vi "ER2007 Test Definition Panel.vi"() -> ()   [LabVIEW 2013]
uses:
  Controls/Global ER2007.vi
panel:
  in  "4P/2P":u16(ring) items=["2-Pole", "4-Pole"]
  in  "ZeroPore":bool
  in  "PoreXdcr":enum16{"Lo Range", "Hi Range"}(ring)
  in  "Volume Measurement":u16(ring) items=["VPA", "Manual"]
  out "NewData":bool
  in  "Stop":bool
  in  "Rw_Temp":dbl=23.0 caption="°C" min=-100.0 format="%.1f"
  in  "Rw":dbl min=0.0 format="%.3f"
  out "Cell ID":string="<none>"
  in  "DAQ Units":u16(ring) items=["Mins", "Hrs"]
  in  "File":path
  in  "Acquisition Period":dbl=60.0 min=1.0
  in  "Frequency (Hz)":dbl=1000.0 min=20.0 max=100000.0
  in  "Electrode Spacing":dbl min=0.0 format="%.3f"
  in  "Permeability":dbl format="%.1f"
  in  "Porosity":dbl format="%.1f"
  in  "Diameter":dbl min=0.0 format="%.3f"
  in  "Length":dbl min=0.0 format="%.3f"
  in  "Fluid Pair":string
  in  "Rock Type":string
  in  "Sample ID":string
  in  "Project":string
  in  "Cancel":bool
  in  "Clear":bool
  in  "Start":bool
  in  "Exit":bool
  # "Test Definition"
  # "Test Description"
  # "Sample Properties"
  # "Project"
  # "Length (cm)"
  # "Sample ID"
  # "Diameter (cm)"
  # "Rock Type"
  # "Porosity (%)"
  # "Fluid Pair"
  # "Permeability (mD)"
  # "Rw"
  # "@"
  # "Electrode Spacing (cm)"
  # "°C"
  # "Test Parameters"
  # "Frequency (Hz)"
  # "Pore Transducer"
  # "Volume Measurement"
  # "Measurement Type"
  # "File"
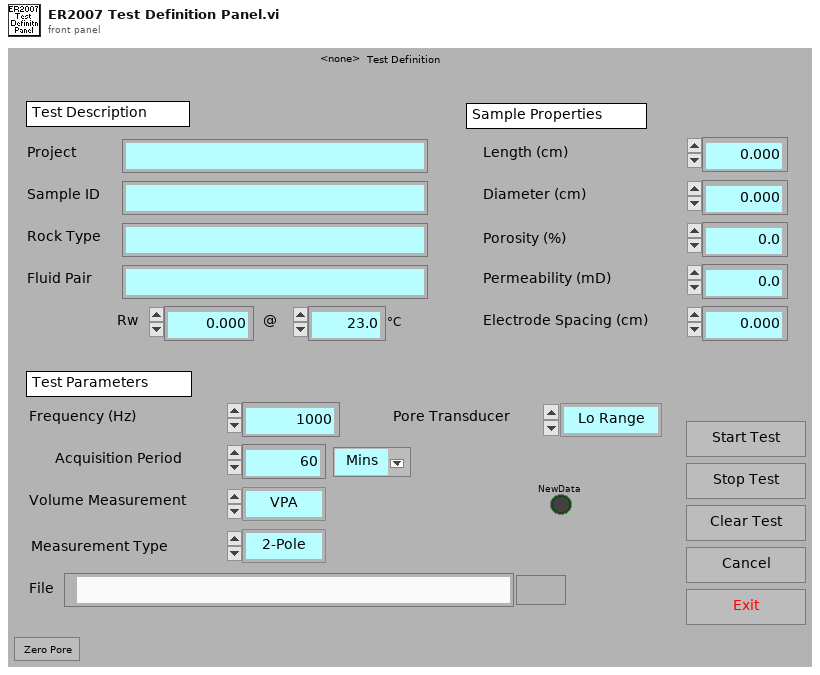
[diagram p1: front panel]
types:
  T1 = enum32{"existing file", "new file", "new or existing file", "existing dir", "new dir", "new or existing dir", "existing file (use LLBs)", "new file (use LLBs)", "new or existing file (use LLBs)", "new or existing file or directory (use LLBs)"}
  T2 = cluster{"CurCell":i32, "Cell Data":cluster{"Cell ID":i32, "Cell Status":enum16{"Inactive", "Setup", "Active", "Done"}, "Project":string, "Sample #":string, "Rock Type":string, "Fluid Pair":string, "Rw":dbl, "Rw Temp":dbl, "Length":dbl, "Diameter":dbl, "Porosity":dbl, "Permeability":dbl, "4P":bool, "ElectSpace":dbl, "Frequency":dbl, "Amplitude":dbl, "DAQ Period":u32, "DAQ Units":u16, "Start Time":dbl, "Next Time":dbl, "Datafile":path, "Last Pore Vol":dbl, "Last Pore Xdcr":enum16{"<none>", "Lo Range", "Hi Range"}, "Last Resistor":enum16{"<none>", "Resistor 1", "Resistor 2", "Resistor 3", "Resistor 4", "Resistor 5", "Resistor 6"}, "CurData":dbl[][], "Comment":string}[]}
  T3 = cluster{"Cell ID":i32, "Cell Status":enum16{"Inactive", "Setup", "Active", "Done"}, "Project":string, "Sample #":string, "Rock Type":string, "Fluid Pair":string, "Rw":dbl, "Rw Temp":dbl, "Length":dbl, "Diameter":dbl, "Porosity":dbl, "Permeability":dbl, "4P":bool, "ElectSpace":dbl, "Frequency":dbl, "Amplitude":dbl, "DAQ Period":u32, "DAQ Units":u16, "Start Time":dbl, "Next Time":dbl, "Datafile":path, "Last Pore Vol":dbl, "Last Pore Xdcr":enum16{"<none>", "Lo Range", "Hi Range"}, "Last Resistor":enum16{"<none>", "Resistor 1", "Resistor 2", "Resistor 3", "Resistor 4", "Resistor 5", "Resistor 6"}, "CurData":dbl[][], "Comment":string}[]
  T4 = cluster{"Cell ID":i32, "Cell Status":enum16{"Inactive", "Setup", "Active", "Done"}, "Project":string, "Sample #":string, "Rock Type":string, "Fluid Pair":string, "Rw":dbl, "Rw Temp":dbl, "Length":dbl, "Diameter":dbl, "Porosity":dbl, "Permeability":dbl, "4P":bool, "ElectSpace":dbl, "Frequency":dbl, "Amplitude":dbl, "DAQ Period":u32, "DAQ Units":u16, "Start Time":dbl, "Next Time":dbl, "Datafile":path, "Last Pore Vol":dbl, "Last Pore Xdcr":enum16{"<none>", "Lo Range", "Hi Range"}, "Last Resistor":enum16{"<none>", "Resistor 1", "Resistor 2", "Resistor 3", "Resistor 4", "Resistor 5", "Resistor 6"}, "CurData":dbl[][], "Comment":string}
  T5 = cluster{"PageTitle":string, "NumLines":i32, "ChlNum":string[], "ChlDesc":string[], "ChlUnits":string[], "ChlZero":sgl[], "ChlFactor":sgl[], "ChlConfig":u16[]}[]
  T6 = cluster{"PageTitle":string, "NumLines":i32, "ChlNum":string[], "ChlDesc":string[], "ChlUnits":string[], "ChlZero":sgl[], "ChlFactor":sgl[], "ChlConfig":u16[]}
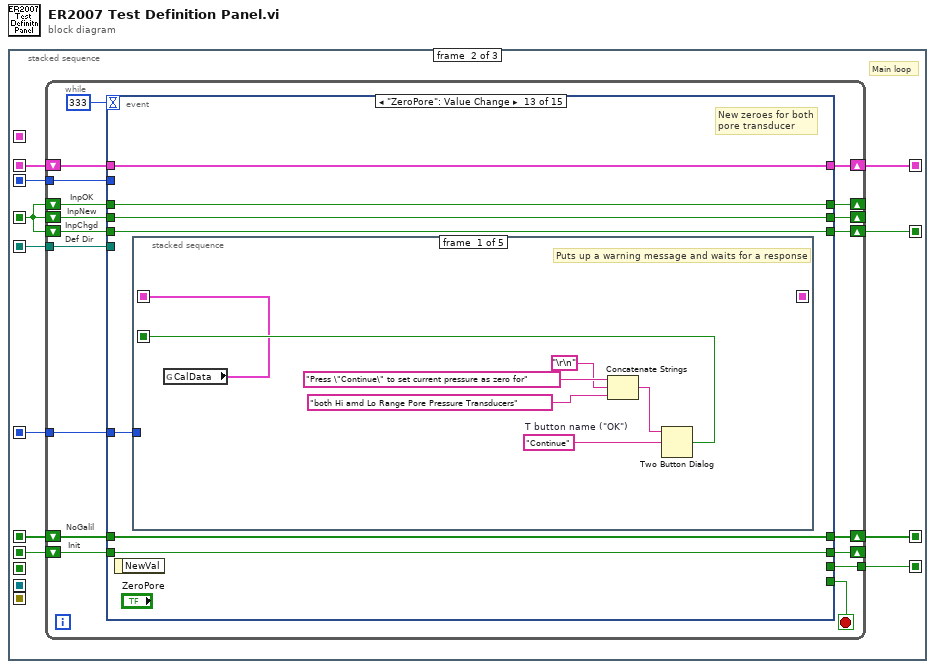
[diagram p0: block diagram]
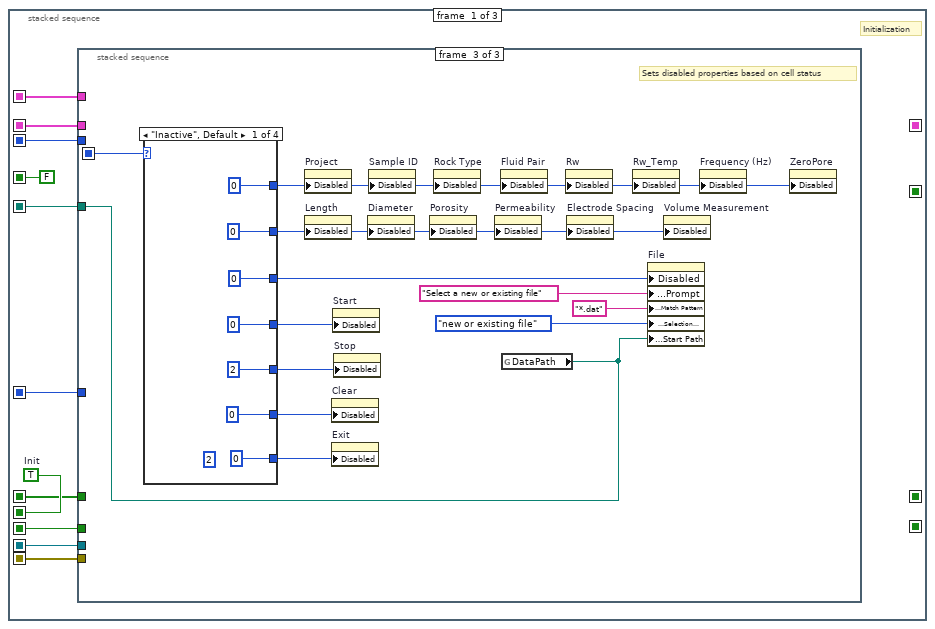
[diagram p2: hidden frame]
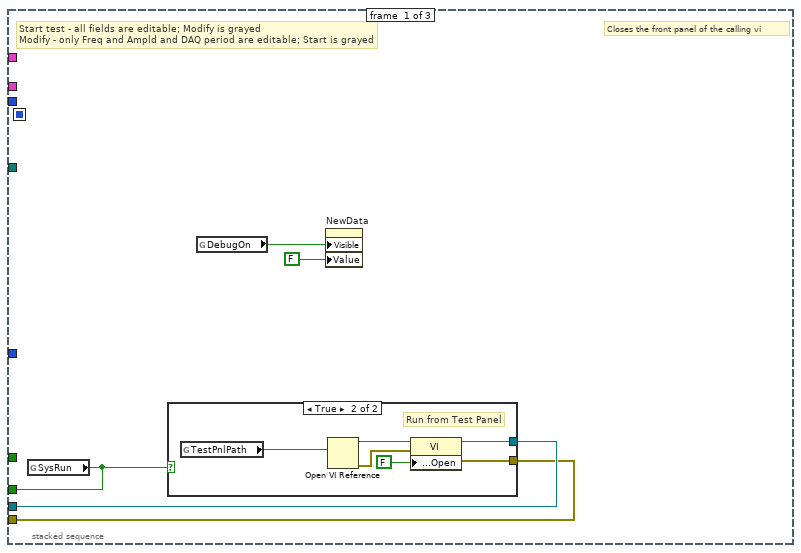
[diagram p3: hidden frame]
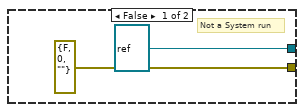
[diagram p4: hidden frame]
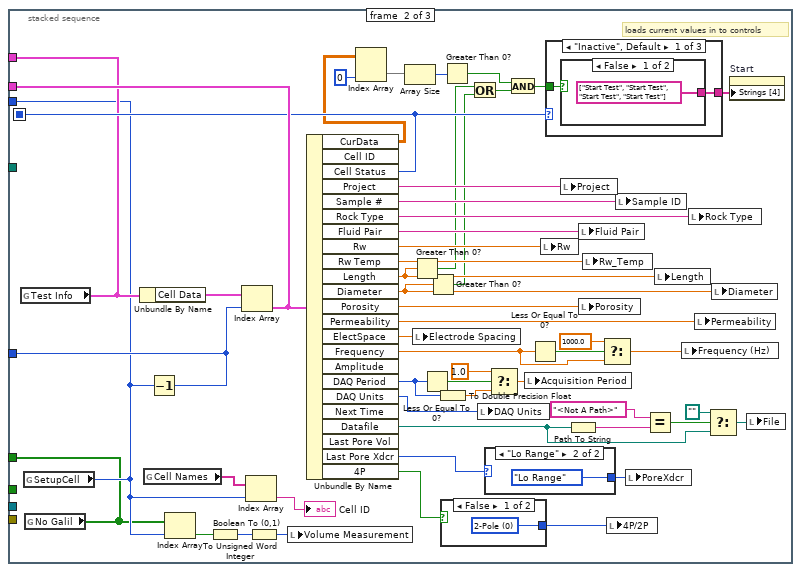
[diagram p5: hidden frame]
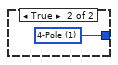
[diagram p6: hidden frame]
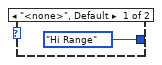
[diagram p7: hidden frame]
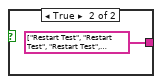
[diagram p8: hidden frame]
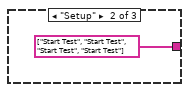
[diagram p9: hidden frame]
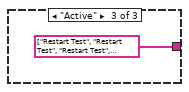
[diagram p10: hidden frame]
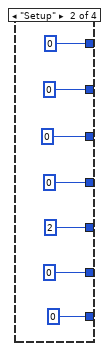
[diagram p11: hidden frame]
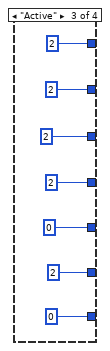
[diagram p12: hidden frame]
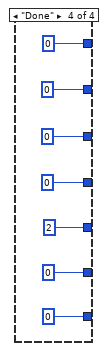
[diagram p13: hidden frame]
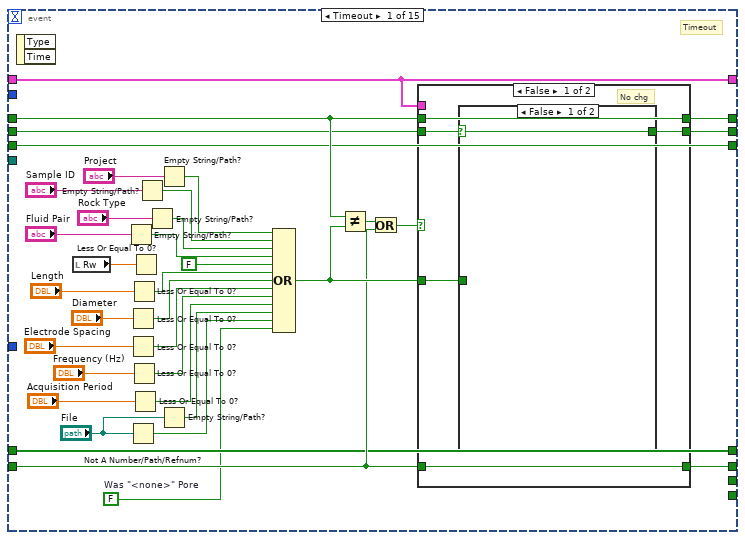
[diagram p14: hidden frame]
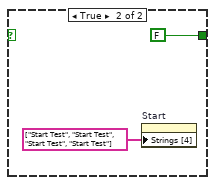
[diagram p15: hidden frame]
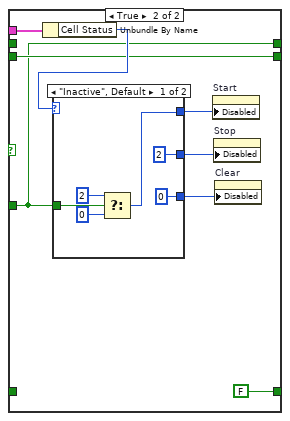
[diagram p16: hidden frame]
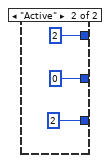
[diagram p17: hidden frame]
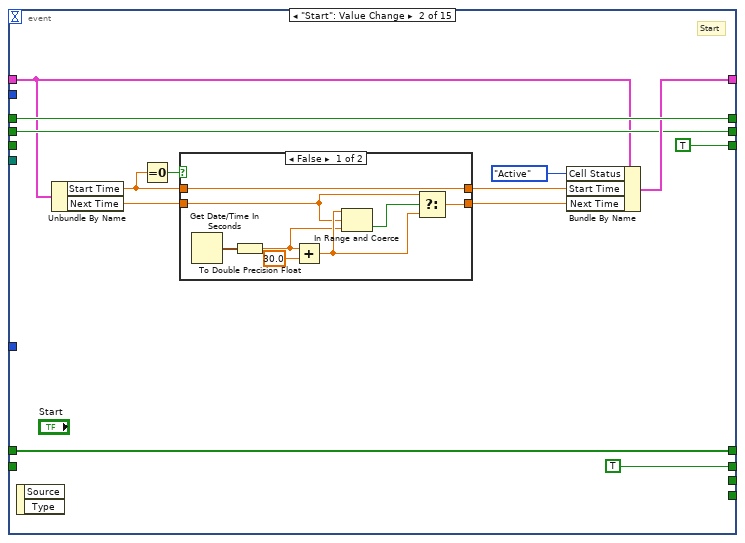
[diagram p18: hidden frame]
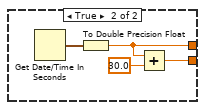
[diagram p19: hidden frame]
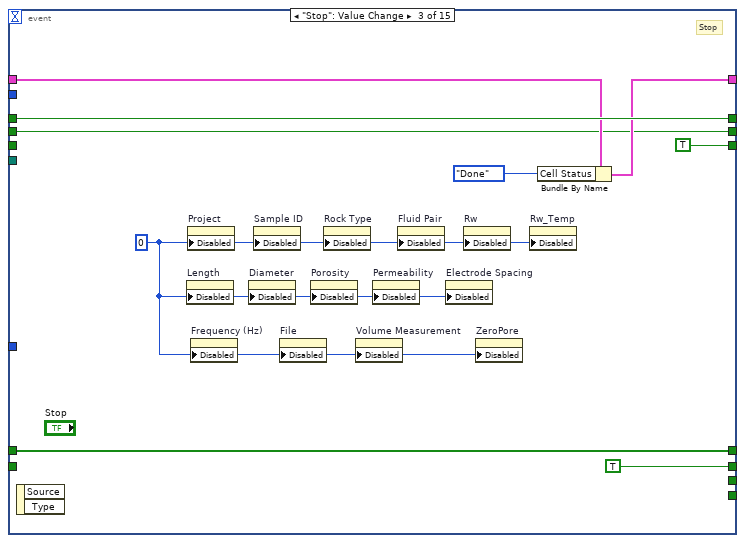
[diagram p20: hidden frame]
diagram:
  n1 = stacked-sequence {
    seq-local: [w11 _ _] -> [_ _ w495]
    seq-local: [_ w138 _] -> [_ _ w494]
    seq-local: [w10 _ _] -> [_ _ _]
    seq-local: [w9 _ _] -> [_ w136 _]
    seq-local: [w7 _ _] -> [_ w131 w493]
    seq-local: [w8 _ _] -> [_ w129 w492]
    seq-local: [w6 _ _] -> [_ _ w490]
    seq-local: [w5 _ _] -> [_ _ w491]
    seq-local: [w4 _ _] -> [_ w137 _]
    seq-local: [_ w135 _] -> [_ _ w489]
    seq-local: [_ w134 _] -> [_ _ w488]
    seq-local: [FALSE _ _] -> [_ w133 _]
    seq-local: [w2 _ _] -> [_ w132 _]
    seq-local: [w1 _ _] -> [_ w130 w487]
    seq-local: [_ w128 _] -> [_ _ w486]
    frame #0 {
      w4 = TRUE  # Init
      # "Initialization"
      n2 = stacked-sequence {
        seq-local: [_ w50 _] -> [_ _ w99]
        tunnel: [w13 _ _] -> w11
        tunnel: [_ w37 _] -> w10
        tunnel: [_ w77 _] -> w9
        tunnel: [_ w33 _] -> w8
        tunnel: [_ w34 _] -> w7
        tunnel: [w16 _ _] -> w6
        tunnel: [w15 _ _] -> w5
        tunnel: [_ _ w90] -> w2
        tunnel: [_ w29 _] -> w1
        frame #0 {
          # "Closes the front panel of the calling vi"
          # "Start test - all fields are editable; Modify is grayed\nModify - only Freq and Ampld and DAQ period are editable; Start is grayed"
          n3 = global read "Global ER2007.vi" "SysRun"() -> (w13:bool)
          n4 = case shown="True" w13 {
            tunnel: [refnum<vi> refnum w21] -> w16
            tunnel: [errorcluster {"status"=FALSE, "code"=0, "source"=""} ("error out") w20] -> w15
            frame False {
              # "Not a System run"
            }
            frame True {
              # "Run from Test Panel"
              n5 = global read "Global ER2007.vi" "TestPnlPath"() -> (w19:path)
              n6 = Open VI Reference(vi path=w19) -> (vi reference=w24:refnum<vi>, error out=w23:errorcluster)  [unwired: 5 in]
              n7 = property class="VI"(reference=w24, error in=w23, "Front Panel Window:Open"=FALSE) -> (reference out=w21:refnum<vi>, error out=w20:errorcluster)
            }
          }
          n8 = global read "Global ER2007.vi" "DebugOn"() -> (w12:bool)
          n9 = property on="NewData" class="Bool (strict)"("Visible"=w12, "Value"=FALSE ("NewData")) -> ()  [unwired: 2 in, 2 out]
        }
        frame #1 {
          # "loads current values in to controls"
          n10 = global read "Global ER2007.vi" "Test Info"() -> (w37:T2)
          n11 = global read "Global ER2007.vi" "SetupCell"() -> (w33:i32)
          n12 = global read "Global ER2007.vi" "No Galil"() -> (w29:bool[])
          n13 = Unbundle By Name(w37) -> ("Cell Data"=w68:T3)
          n14 = global read "Global ER2007.vi" "Cell Names"() -> (w36:string[])
          n15 = Decrement(x=w33) -> (x-1=w34:i32)
          n16 = Index Array(array=w29, index=w33) -> (element=w32:bool)
          n17 = Boolean To (0,1)(Boolean=w32) -> (0, 1=w31:i16)
          n18 = Index Array(array=w68, index=w34) -> (element=w77:T4)
          n19 = Index Array(array=w36, index=w33) -> (element=→"Cell ID":string)
          n20 = To Unsigned Word Integer(number=w31) -> (unsigned 16bit integer=w30:u16)
          n21 = local write "Volume Measurement"(w30) -> ()
          n22 = Unbundle By Name(w77) -> ("CurData"=w44:dbl[][], "Cell Status"=w50:enum16{"Inactive", "Setup", "Active", "Done"}, "Project"=w76:string, "Sample #"=w75:string, "Rock Type"=w74:string, "Fluid Pair"=w73:string, "Rw"=w67:dbl, "Rw Temp"=w66:dbl, "Length"=w48:dbl, "Diameter"=w47:dbl, "Porosity"=w72:dbl, "Permeability"=w71:dbl, "ElectSpace"=w70:dbl, "Frequency"=w59:dbl, "DAQ Period"=w65:u32, "DAQ Units"=w69:u16, "Datafile"=w53:path, "Last Pore Xdcr"=w27:enum16{"<none>", "Lo Range", "Hi Range"}, "4P"=w26:bool)  [unwired: 4 out]
          n23 = Index Array(array=w44, index (col)=0 ("disabled index (col)")) -> (element=w42:dbl[])  [unwired: 1 in]
          n24 = Array Size(array=w42) -> (size(s)=w39:i32)
          n25 = Greater Than 0?(x=w48) -> (x > 0?=w46:bool)
          n26 = local write "Electrode Spacing"(w70) -> ()
          n27 = Less Or Equal To 0?(x=w65) -> (x <= 0?=w64:bool)
          n28 = Greater Than 0?(x=w47) -> (x > 0?=w45:bool)
          n29 = To Double Precision Float(number=w65) -> (double precision float=w63:dbl)
          n30 = case shown="False" w26 {
            tunnel: [w78 w79] -> w25
            frame False {
              w78 = u16 0 items=["2-Pole", "4-Pole"] ("4P/2P")
            }
            frame True {
              w79 = u16 1 items=["2-Pole", "4-Pole"] ("4P/2P")
            }
          }
          n31 = Greater Than 0?(x=w39) -> (x > 0?=w38:bool)
          n32 = Or(x=w46, y=w45) -> (x .or. y?=w40:bool)
          n33 = local write "DAQ Units"(w69) -> ()
          n34 = case shown="\"Lo Range\"" w27 {
            tunnel: [enum16{"Lo Range", "Hi Range"}."Hi Range" ("PoreXdcr") enum16{"Lo Range", "Hi Range"}."Lo Range" ("PoreXdcr")] -> w28
            frame "<none>", Default {
            }
            frame "Lo Range" {
            }
          }
          n35 = Select(t=1.0, s=w64, f=w63) -> (s? t:f=w62:dbl)
          n36 = And(x=w38, y=w40) -> (x .and. y?=w41:bool)
          n37 = local write "Acquisition Period"(w62) -> ()
          n38 = Less Or Equal To 0?(x=w59) -> (x <= 0?=w60:bool)
          n39 = local write "Rw"(w67) -> ()
          n40 = case shown="\"Inactive\", Default" w50 {
            tunnel: [w83 string[] ["Start Test", "Start Test", "Start Test", "Start Test"] ("Strings [4]") string[] ["Restart Test", "Restart Test", "Restart Test", "Restart Test"] ("Strings [4]")] -> w49
            tunnel: w41 -> [w82 _ _]
            frame "Inactive", Default {
              n41 = case shown="False" w82 {
                tunnel: [string[] ["Start Test", "Start Test", "Start Test", "Start Test"] ("Strings [4]") string[] ["Restart Test", "Restart Test", "Restart Test", "Restart Test"] ("Strings [4]")] -> w83
                frame False {
                }
                frame True {
                }
              }
            }
            frame "Setup" {
            }
            frame "Active" {
            }
          }
          n42 = local write "Project"(w76) -> ()
          n43 = Path To String(path=w53) -> (string=w55:string)
          n44 = local write "Fluid Pair"(w73) -> ()
          n45 = local write "Porosity"(w72) -> ()
          n46 = local write "Rw_Temp"(w66) -> ()
          n47 = Select(t=1000.0, s=w60, f=w59) -> (s? t:f=w58:dbl)
          n48 = local write "4P/2P"(w25) -> ()
          n49 = local write "Sample ID"(w75) -> ()
          n50 = local write "PoreXdcr"(w28) -> ()
          n51 = Equal?(x="<Not A Path>" ("y"), y=w55) -> (x = y?=w56:bool)
          n52 = local write "Length"(w48) -> ()
          n53 = local write "Frequency (Hz)"(w58) -> ()
          n54 = local write "Rock Type"(w74) -> ()
          n55 = local write "Permeability"(w71) -> ()
          n56 = Select(t=path "", s=w56, f=w53) -> (s? t:f=w52:path)
          n57 = local write "Diameter"(w47) -> ()
          n58 = property on="Start" class="Bool"("Strings [4]"=w49) -> ()  [unwired: 2 in, 2 out]
          n59 = local write "File"(w52) -> ()
        }
        frame #2 {
          # "Sets disabled properties based on cell status"
          n60 = case shown="\"Inactive\", Default" w99 {
            tunnel: [u8 0 ("Disabled") u8 0 ("Disabled") u8 2 ("Disabled") u8 0 ("Disabled")] -> w89
            tunnel: [u8 0 ("Disabled") u8 0 ("Disabled") u8 2 ("Disabled") u8 0 ("Disabled")] -> w88
            tunnel: [u8 0 ("Disabled") u8 0 ("Disabled") u8 2 ("Disabled") u8 0 ("Disabled")] -> w98
            tunnel: [u8 0 ("Disabled") u8 0 ("Disabled") u8 2 ("Disabled") u8 0 ("Disabled")] -> w97
            tunnel: [u8 0 ("Disabled") u8 0 ("Disabled") u8 2 ("Disabled") u8 0 ("Disabled")] -> w96
            tunnel: [u8 2 ("Disabled") u8 2 ("Disabled") u8 0 ("Disabled") u8 2 ("Disabled")] -> w95
            tunnel: [u8 0 ("Disabled") u8 0 ("Disabled") u8 0 ("Disabled") u8 0 ("Disabled")] -> w94
            frame "Inactive", Default {
              (unwired) u8 2 ("Disabled")
            }
            frame "Setup" {
            }
            frame "Active" {
            }
            frame "Done" {
            }
          }
          n61 = property on="Project" class="Str"("Disabled"=w89) -> ()  [unwired: 2 in, 2 out]
          n62 = property on="Length" class="DigNum (strict)"("Disabled"=w88) -> ()  [unwired: 2 in, 2 out]
          n63 = property on="Clear" class="Bool"("Disabled"=w97) -> ()  [unwired: 2 in, 2 out]
          n64 = property on="Exit" class="Bool"("Disabled"=w94) -> ()  [unwired: 2 in, 2 out]
          n65 = property on="Start" class="Bool"("Disabled"=w98) -> ()  [unwired: 2 in, 2 out]
          n66 = property on="Stop" class="Bool"("Disabled"=w95) -> ()  [unwired: 2 in, 2 out]
          n67 = property on="Diameter" class="DigNum (strict)"("Disabled"=w88) -> ()  [unwired: 2 in, 2 out]
          n68 = property on="Sample ID" class="Str"("Disabled"=w89) -> ()  [unwired: 2 in, 2 out]
          n69 = property on="Porosity" class="DigNum (strict)"("Disabled"=w88) -> ()  [unwired: 2 in, 2 out]
          n70 = property on="Rock Type" class="Str"("Disabled"=w89) -> ()  [unwired: 2 in, 2 out]
          n71 = property on="Permeability" class="DigNum (strict)"("Disabled"=w88) -> ()  [unwired: 2 in, 2 out]
          n72 = property on="Fluid Pair" class="Str"("Disabled"=w89) -> ()  [unwired: 2 in, 2 out]
          n73 = global read "Global ER2007.vi" "DataPath"() -> (w90:path)
          n74 = property on="Rw" class="DigNum (strict)"("Disabled"=w89) -> ()  [unwired: 2 in, 2 out]
          n75 = property on="Electrode Spacing" class="DigNum (strict)"("Disabled"=w88) -> ()  [unwired: 2 in, 2 out]
          n76 = property on="Rw_Temp" class="DigNum (strict)"("Disabled"=w89) -> ()  [unwired: 2 in, 2 out]
          n77 = property on="File" class="Path"("Disabled"=w96, "Browse Options:Prompt"="Select a new or existing file" ("Browse Dialog Options:Prompt"), "Browse Options:Match Pattern"="*.dat" ("Browse Dialog Options:Match Pattern"), "Browse Options:Selection Mode"=T1."new or existing file" ("Browse Dialog Options:Selection Mode"), "Browse Options:Start Path"=w90) -> ()  [unwired: 2 in, 2 out]
          n78 = property on="Volume Measurement" class="Ring (strict)"("Disabled"=w88) -> ()  [unwired: 2 in, 2 out]
          n79 = property on="Frequency (Hz)" class="DigNum (strict)"("Disabled"=w89) -> ()  [unwired: 2 in, 2 out]
          n80 = property on="ZeroPore" class="Bool"("Disabled"=w89) -> ()  [unwired: 2 in, 2 out]
        }
      }
    }
    frame #1 {
      # "Main loop"
      n81 = while {
        tunnel: [w154] -> w138
        shift-right: [w152] -> _
        shift-left: w133 -> [w153]
        shift-right: [w150] -> _
        shift-left: w137 -> [w151]
        shift-right: [w148] -> w135
        shift-left: w136 -> [w149]
        shift-right: [w146] -> _
        shift-left: w133 -> [w147]
        shift-right: [w144] -> w134
        shift-left: w133 -> [w145]
        tunnel: w132 -> [w143]
        tunnel: w131 -> [w142]
        shift-right: [w140] -> w128
        shift-left: w130 -> [w141]
        tunnel: w129 -> [w139]
        stop <- w155 stop-if-true
        # "Init"
        # "NoGalil"
        # "Def Dir"
        # "InpNew"
        # "InpOK"
        # "InpChgd"
        n82 = event shown="[12] \"ZeroPore\": Value Change" {
          selector: _ -> [_ _ _ _ _ _ _ _ _ _ _ _ _ _ _]
          dyn-events: _ -> [_ _ _ _ _ _ _ _ _ _ _ _ _ _ _]
          timeout: 333 -> [_ _ _ _ _ _ _ _ _ _ _ _ _ _ _]
          tunnel: [_ _ _ _ _ _ _ _ _ _ _ _ _ w460 w464] -> w155
          tunnel: [_ _ _ _ _ _ _ _ _ _ _ _ _ FALSE w464] -> w154
          tunnel: w153 -> [w185 w230 w251 w274 w281 w287 w294 w299 w309 w315 w337 w381 w389 w458 w465]
          tunnel: [w183 w230 w251 w274 w281 w287 w294 w299 w309 w315 w337 w381 w389 w458 w465] -> w152
          tunnel: w151 -> [w162 _ _ _ w279 w285 w291 w296 w307 w311 w339 w377 w385 w457 w468]
          tunnel: [w163 TRUE ("Init") TRUE ("Init") TRUE ("Init") w279 w285 w291 w296 w307 w311 w339 w377 w385 w457 w468] -> w150
          tunnel: w149 -> [w181 w223 w249 _ w282 w288 w293 w300 w310 w316 w338 w382 w384 w456 w467]
          tunnel: [w181 w228 w248 w256 w282 w288 w293 w300 w310 w316 w338 w382 w384 w456 w467] -> w148
          tunnel: w147 -> [w161 w224 w246 _ _ _ _ w298 _ _ _ w380 w388 w455 w466]
          tunnel: [w160 w224 w246 TRUE TRUE TRUE TRUE w298 TRUE FALSE TRUE w380 w388 w455 w466] -> w146
          tunnel: w145 -> [w159 _ _ _ _ _ _ _ _ _ _ _ w387 _ w463]
          tunnel: [w159 TRUE TRUE TRUE TRUE TRUE TRUE TRUE TRUE TRUE TRUE TRUE w387 FALSE w463] -> w144
          tunnel: w143 -> [_ _ _ _ _ _ _ _ _ _ w322 _ _ _ _]
          tunnel: w142 -> [_ _ _ _ _ _ _ _ _ _ w318 _ w383 _ _]
          tunnel: w141 -> [w158 w218 w244 w253 w277 w283 w289 w295 w306 w312 w317 w378 w386 w453 w461]
          tunnel: [w158 w218 w244 w253 w277 w283 w289 w295 w305 w312 w317 w378 w386 w453 w461] -> w140
          tunnel: w139 -> [_ _ _ _ _ _ _ _ w304 _ _ _ _ _ _]
          event Timeout {
            w157 = FALSE  # Was "<none>" Pore
            # "Timeout"
            n83 = event-data() -> ()  [unwired: 1 in, 2 out]
            n84 = local read "Rw"() -> (w164:dbl)
            n85 = Empty String/Path?(string/path="Fluid Pair") -> (empty?=w189:bool)
            n86 = Less Or Equal To 0?(x="Diameter") -> (x <= 0?=w187:bool)
            n87 = Less Or Equal To 0?(x="Electrode Spacing") -> (x <= 0?=w186:bool)
            n88 = Not A Number/Path/Refnum?(number/path/refnum="File") -> (NaN/Path/Refnum?=w179:bool)
            n89 = Less Or Equal To 0?(x="Length") -> (x <= 0?=w188:bool)
            n90 = Less Or Equal To 0?(x="Frequency (Hz)") -> (x <= 0?=w177:bool)
            n91 = Less Or Equal To 0?(x="Acquisition Period") -> (x <= 0?=w168:bool)
            n92 = Less Or Equal To 0?(x=w164) -> ()  [unwired: 1 out]
            n93 = Empty String/Path?(string/path="Sample ID") -> (empty?=w191:bool)
            n94 = Empty String/Path?(string/path="Rock Type") -> (empty?=w190:bool)
            n95 = Empty String/Path?(string/path="Project") -> (empty?=w192:bool)
            n96 = Empty String/Path?(string/path="File") -> (empty?=w178:bool)
            n97 = Compound Arithmetic op=OR(w192, w191, w190, w189, FALSE ("value"), w188, w187, w186, w177, w168, w178, w179, w157) -> (w180:bool)
            n98 = Not Equal?(x=w185, y=w180) -> (x != y?=w184:bool)
            n99 = Or(x=w184, y=w162) -> (x .or. y?=w182:bool)
            n100 = case shown="False" w182 {
              tunnel: w185 -> [w197 _]
              tunnel: [w197 w201] -> w183
              tunnel: w180 -> [w193 w201]
              tunnel: w181 -> [_ w208]
              tunnel: [w196 FALSE ("Init")] -> w163
              tunnel: w162 -> [w196 _]
              tunnel: w161 -> [w195 w202]
              tunnel: [w194 w202] -> w160
              frame False {
                # "No chg"
                n101 = case shown="False" w195 {
                  selector: w195 -> [w198 _]
                  tunnel: [w198 FALSE] -> w194
                  tunnel: w193 -> [_ _]
                  frame False {
                  }
                  frame True {
                    n102 = property on="Start" class="Bool"("Strings [4]"=string[] ["Start Test", "Start Test", "Start Test", "Start Test"]) -> ()  [unwired: 2 in, 2 out]
                  }
                }
              }
              frame True {
                n103 = Unbundle By Name(w208) -> ("Cell Status"=w207:enum16{"Inactive", "Setup", "Active", "Done"})
                n104 = case shown="\"Inactive\", Default" w207 {
                  tunnel: [u8 2 ("Disabled") u8 0 ("Disabled")] -> w206
                  tunnel: [w209 u8 2 ("Disabled")] -> w205
                  tunnel: [u8 0 ("Disabled") u8 2 ("Disabled")] -> w204
                  tunnel: w201 -> [w210 _]
                  frame "Inactive", Default {
                    n105 = Select(t=u8 2 ("Disabled"), s=w210, f=u8 0 ("Disabled")) -> (s? t:f=w209:u8)
                  }
                  frame "Active" {
                  }
                }
                n106 = property on="Start" class="Bool"("Disabled"=w205) -> ()  [unwired: 2 in, 2 out]
                n107 = property on="Stop" class="Bool"("Disabled"=w206) -> ()  [unwired: 2 in, 2 out]
                n108 = property on="Clear" class="Bool"("Disabled"=w204) -> ()  [unwired: 2 in, 2 out]
              }
            }
          }
          event "Start": Value Change {
            # "Start"
            n109 = event-data() -> ()  [unwired: 1 in, 2 out]
            n110 = Unbundle By Name(w223) -> ("Start Time"=w221:dbl, "Next Time"=w222:dbl)
            n111 = Equal To 0?(x=w221) -> (x = 0?=w219:bool)
            n112 = case shown="False" w219 {
              tunnel: [w236 w240] -> w226
              tunnel: [w238 w239] -> w225
              tunnel: w222 -> [w232 _]
              tunnel: w221 -> [w238 _]
              frame False {
                n113 = Get Date/Time In Seconds() -> (seconds since 1Jan1904=w237:timestamp)
                n114 = To Double Precision Float(number=w237) -> (double precision float=w233:dbl)
                n115 = Add(x=w233, y=30.0) -> (x+y=w234:dbl)
                n116 = In Range and Coerce(upper limit=w234, x=w232, lower limit=w233) -> (In Range?=w231:bool)  [unwired: 1 out]
                n117 = Select(t=w232, s=w231, f=w234) -> (s? t:f=w236:dbl)
              }
              frame True {
                n118 = Get Date/Time In Seconds() -> (seconds since 1Jan1904=w242:timestamp)
                n119 = To Double Precision Float(number=w242) -> (double precision float=w239:dbl)
                n120 = Add(x=w239, y=30.0) -> (x+y=w240:dbl)
              }
            }
            n121 = Bundle By Name(cluster=w223, "Cell Status"=enum16{"Inactive", "Setup", "Active", "Done"}."Active", "Start Time"=w225, "Next Time"=w226) -> (w228:T4)
          }
          event "Stop": Value Change {
            w243 = u8 0 ("Disabled")
            # "Stop"
            n122 = event-data() -> ()  [unwired: 1 in, 2 out]
            n123 = property on="Length" class="DigNum (strict)"("Disabled"=w243) -> ()  [unwired: 2 in, 2 out]
            n124 = property on="Project" class="Str"("Disabled"=w243) -> ()  [unwired: 2 in, 2 out]
            n125 = property on="Frequency (Hz)" class="DigNum (strict)"("Disabled"=w243) -> ()  [unwired: 2 in, 2 out]
            n126 = property on="Diameter" class="DigNum (strict)"("Disabled"=w243) -> ()  [unwired: 2 in, 2 out]
            n127 = property on="Sample ID" class="Str"("Disabled"=w243) -> ()  [unwired: 2 in, 2 out]
            n128 = property on="File" class="Path"("Disabled"=w243) -> ()  [unwired: 2 in, 2 out]
            n129 = property on="Porosity" class="DigNum (strict)"("Disabled"=w243) -> ()  [unwired: 2 in, 2 out]
            n130 = property on="Rock Type" class="Str"("Disabled"=w243) -> ()  [unwired: 2 in, 2 out]
            n131 = property on="Volume Measurement" class="Ring (strict)"("Disabled"=w243) -> ()  [unwired: 2 in, 2 out]
            n132 = property on="Permeability" class="DigNum (strict)"("Disabled"=w243) -> ()  [unwired: 2 in, 2 out]
            n133 = property on="Fluid Pair" class="Str"("Disabled"=w243) -> ()  [unwired: 2 in, 2 out]
            n134 = property on="Electrode Spacing" class="DigNum (strict)"("Disabled"=w243) -> ()  [unwired: 2 in, 2 out]
            n135 = property on="Rw" class="DigNum (strict)"("Disabled"=w243) -> ()  [unwired: 2 in, 2 out]
            n136 = property on="ZeroPore" class="Bool"("Disabled"=w243) -> ()  [unwired: 2 in, 2 out]
            n137 = property on="Rw_Temp" class="DigNum (strict)"("Disabled"=w243) -> ()  [unwired: 2 in, 2 out]
            n138 = Bundle By Name(cluster=w249, "Cell Status"=enum16{"Inactive", "Setup", "Active", "Done"}."Done") -> (w248:T4)
          }
          event "Clear": Value Change {
            w256 = T4 {"Cell ID"=0, "Cell Status"=enum."Inactive", "Project"="", "Sample #"="", "Rock Type"="", "Fluid Pair"="", "Rw"=0.0, "Rw Temp"=0.0, "Length"=0.0, "Diameter"=0.0, "Porosity"=0.0, "Permeability"=0.0, "4P"=TRUE, "ElectSpace"=0.0, "Frequency"=0.0, "Amplitude"=0.0, "DAQ Period"=0, "DAQ Units"=0, "Start Time"=0.0, "Next Time"=0.0, "Datafile"=path "", "Last Pore Vol"=0.0, "Last Pore Xdcr"=enum."<none>", "Last Resistor"=enum."<none>", "CurData"=[], "Comment"=""} ("Cell x Data")
            w255 = u8 0 ("Disabled")
            # "Clear"
            n139 = event-data() -> ()  [unwired: 1 in, 2 out]
            n140 = Unbundle By Name(w256) -> ("Project"=w272:string, "Sample #"=w271:string, "Rock Type"=w270:string, "Fluid Pair"=w269:string, "Rw"=w268:dbl, "Rw Temp"=w267:dbl, "Length"=w266:dbl, "Diameter"=w265:dbl, "Porosity"=w264:dbl, "Permeability"=w263:dbl, "ElectSpace"=w262:dbl, "Datafile"=w259:path, "4P"=w254:bool)
            n141 = case shown="False" w254 {
              tunnel: [w275 w276] -> w252
              frame False {
                w275 = u16 0 items=["2-Pole", "4-Pole"] ("4P/2P")
              }
              frame True {
                w276 = u16 1 items=["2-Pole", "4-Pole"] ("4P/2P")
              }
            }
            n142 = global write "Global ER2007.vi" "SUP Cleared"(TRUE ("SUP Cleared")) -> ()
            n143 = local write "4P/2P"(w252) -> ()
            n144 = property on="Project" class="Str"("Disabled"=w255, "Value"=w272) -> ()  [unwired: 2 in, 2 out]
            n145 = property on="Rw" class="DigNum (strict)"("Disabled"=w255, "Value"=w268) -> ()  [unwired: 2 in, 2 out]
            n146 = property on="Porosity" class="DigNum (strict)"("Disabled"=w255, "Value"=w264) -> ()  [unwired: 2 in, 2 out]
            n147 = property on="Permeability" class="DigNum (strict)"("Disabled"=w255, "Value"=w263) -> ()  [unwired: 2 in, 2 out]
            n148 = property on="Rw_Temp" class="DigNum (strict)"("Disabled"=w255, "Value"=w267) -> ()  [unwired: 2 in, 2 out]
            n149 = property on="File" class="Path"("Disabled"=w255, "Value"=w259) -> ()  [unwired: 2 in, 2 out]
            n150 = property on="Sample ID" class="Str"("Disabled"=w255, "Value"=w271) -> ()  [unwired: 2 in, 2 out]
            n151 = property on="Volume Measurement" class="Ring (strict)"("Disabled"=w255) -> ()  [unwired: 2 in, 2 out]
            n152 = property on="Length" class="DigNum (strict)"("Disabled"=w255, "Value"=w266) -> ()  [unwired: 2 in, 2 out]
            n153 = property on="Electrode Spacing" class="DigNum (strict)"("Disabled"=w255, "Value"=w262) -> ()  [unwired: 2 in, 2 out]
            n154 = property on="Rock Type" class="Str"("Disabled"=w255, "Value"=w270) -> ()  [unwired: 2 in, 2 out]
            n155 = property on="ZeroPore" class="Bool"("Disabled"=w255) -> ()  [unwired: 2 in, 2 out]
            n156 = property on="Frequency (Hz)" class="DigNum (strict)"("Disabled"=w255, "Value"=1000.0 ("Frequency (Hz)")) -> ()  [unwired: 2 in, 2 out]
            n157 = property on="Fluid Pair" class="Str"("Disabled"=w255, "Value"=w269) -> ()  [unwired: 2 in, 2 out]
            n158 = property on="Diameter" class="DigNum (strict)"("Disabled"=w255, "Value"=w265) -> ()  [unwired: 2 in, 2 out]
          }
          event "Project", "Sample ID", "Rock Type", "Fluid Pair", "Rw", "Rw_Temp": Value Change {
            # "Project, etc"
            n159 = event-data() -> ()  [unwired: 1 in, 2 out]
          }
          event "Length", "Diameter", "Porosity", "Permeability", "Electrode Spacing": Value Change {
            # "Length, etc"
            n160 = event-data() -> ()  [unwired: 1 in, 2 out]
          }
          event "Frequency (Hz)": Value Change {
            # "Frequency chgd"
            n161 = event-data() -> ()  [unwired: 1 in, 2 out]
          }
          event "Acquisition Period": Value Change {
            # "Acquisition period chgd"
            n162 = event-data() -> ()  [unwired: 1 in, 2 out]
          }
          event "Volume Measurement": Value Change {
            # "Vol Measurement chgd"
            n163 = event-data() -> ()  [unwired: 1 in, 2 out]
            n164 = Not Equal To 0?(x="Volume Measurement") -> (x != 0?=w302:bool)
            n165 = Replace Array Subset(array=w306, new element=w302, index=w304) -> (w305:bool[])
          }
          event "4P/2P": Value Change {
            # "2-Pole/4-Pole"
            n166 = event-data() -> ()  [unwired: 1 in, 2 out]
          }
          event "File": Value Change {
            w330 = "."  # dot
            w333 = path ""  # dot
            # "File changed - check it\nand fix as necessary"
            n167 = event-data() -> ("NewVal"=w334:path)  [unwired: 1 in]
            n168 = case shown="0, Default" w318 {
              tunnel: ["Cell1.dat" "Cell2.dat" "Cell3.dat" "Cell4.dat" "Cell5.dat"] -> w319
              frame 0, Default {
              }
              frame 1 {
              }
              frame 2 {
              }
              frame 3 {
              }
              frame 4 {
              }
            }
            n169 = Strip Path(path=w334) -> (stripped path=w324:path, name=w323:string)
            n170 = Search/Split String(string=w323, search string/char (-)=w330) -> (substring before match=w327:string, offset of match=w329:i32)  [unwired: 1 in, 1 out]
            n171 = Less Than 0?(x=w329) -> (x < 0?=w328:bool)
            n172 = String Length(string=w323) -> (length=w326:i32)
            n173 = Equal To 0?(x=w329) -> (x = 0?=w325:bool)
            n174 = Equal?(x=w333, y=w324) -> (x = y?=w332:bool)
            n175 = case shown="False" w328 {
              tunnel: w323 -> [w347 _]
              tunnel: w327 -> [_ w359]
              tunnel: w326 -> [w348 w360]
              tunnel: w325 -> [w349 _]
              tunnel: [w346 w358] -> w321
              tunnel: w319 -> [w345 w357]
              frame False {
                n176 = case shown="False" w349 {
                  tunnel: w348 -> [w353 _]
                  tunnel: w347 -> [w352 _]
                  tunnel: [w351 w356] -> w346
                  tunnel: w345 -> [w350 w356]
                  frame False {
                    n177 = case shown="1, Default" w353 {
                      tunnel: w352 -> [_ w355]
                      tunnel: [w354 w355] -> w351
                      tunnel: w350 -> [w354 _]
                      frame 0 {
                        # "No name"
                      }
                      frame 1, Default {
                        # "OK"
                      }
                    }
                  }
                  frame True {
                    # "dot at 1st position"
                  }
                }
              }
              frame True {
                # "No dot"
                n178 = case shown="0" w360 {
                  tunnel: w359 -> [_ w364]
                  tunnel: [w361 w363] -> w358
                  tunnel: w357 -> [w361 _]
                  frame 0 {
                    # "No name either"
                  }
                  frame 1, Default {
                    # "Name but no ext"
                    n179 = Concatenate Strings(w364, ".dat" ("string")) -> (w363:string)
                  }
                }
              }
            }
            n180 = case shown="False" w332 {
              tunnel: w324 -> [w371 _]
              tunnel: [w374 FALSE ("directory")] -> w331
              tunnel: [w372 FALSE ("status")] -> _
              frame False {
                # "Prevents err msg"
                # "TRUE if dir exists"
                n181 = File/Directory Info(path=w371) -> (directory=w374:bool, error out=w373:errorcluster)  [unwired: 1 in, 5 out]
                n182 = Unbundle By Name(w373) -> ("status"=w372:bool)
              }
              frame True {
                # "No dir"
              }
            }
            n183 = case shown="False" w331 {
              tunnel: w324 -> [_ w370]
              tunnel: w321 -> [w367 w369]
              tunnel: w322 -> [w366 _]
              tunnel: [w365 w368] -> w320
              frame False {
                # "Dir does not exist"
                n184 = Build Path(base path=w366, name or relative path=w367) -> (appended path=w365:path)
              }
              frame True {
                # "Dir exists"
                n185 = Build Path(base path=w370, name or relative path=w369) -> (appended path=w368:path)
              }
            }
            n186 = local write "File"(w320) -> ()
          }
          event "PoreXdcr": Value Change {
            # "Active pore xdcr chgd"
            n187 = event-data() -> ()  [unwired: 1 in, 1 out]
          }
          event "ZeroPore": Value Change {
            # "New zeroes for both\npore transducer"
            n188 = event-data() -> ()  [unwired: 1 in, 1 out]
            n189 = stacked-sequence {
              seq-local: [w391 _ _ _ _] -> [_ w399 w446 w449 w451]
              seq-local: [w390 _ _ _ _] -> [_ w398 _ _ _]
              seq-local: [_ w397 _ _ _] -> [_ _ w445 _ _]
              tunnel: w383 -> [_ w400 _ _ _]
              frame #0 {
                w396 = "Continue"  # T button name ("OK")
                # "Puts up a warning message and waits for a response"
                n190 = global read "Global ER2007.vi" "CalData"() -> (w390:T5)
                n191 = Concatenate Strings("Press \"Continue\" to set current pressure as zero for" ("message"), "\r\n", "both Hi amd Lo Range Pore Pressure Transducers" ("message")) -> (w392:string)
                n192 = Two Button Dialog(message=w392, 2:w396) -> (T button?=w391:bool)  [unwired: 1 in]
              }
              frame #1 {
                # "If \"Continue\", updates CalData with new pore zeroes"
                n193 = case shown="True" w399 {
                  tunnel: w400 -> [_ w419]
                  tunnel: w398 -> [w401 w403]
                  tunnel: [w401 w402] -> w397
                  frame False {
                    # "No update"
                  }
                  frame True {
                    # "User wants to update zeroes"
                    n194 = case shown="0, Default" w419 {
                      tunnel: [0 ("index") 1 ("index") 1 ("index") 2 ("index") 2 ("index")] -> w417
                      tunnel: [8 ("index") 8 ("index") 5 ("index") 8 ("index") 5 ("index")] -> w412
                      tunnel: [3 ("index") 3 ("index") 13 ("index") 3 ("index") 13 ("index")] -> w411
                      tunnel: [w421 w426 w431 w436 w441] -> w406
                      tunnel: [w420 w425 w430 w435 w440] -> w405
                      frame 0, Default {
                        w420 = 3  # Hi
                        w421 = 4  # Lo
                        # "Cell 1"
                      }
                      frame 1 {
                        w425 = 10  # HI
                        w426 = 14  # Lo
                        # "Cell 2"
                      }
                      frame 2 {
                        w430 = 18  # Hi
                        w431 = 11  # Lo
                        # "Cell 3"
                      }
                      frame 3 {
                        w435 = 24  # Hi
                        w436 = 28  # Lo
                        # "Cell 4"
                      }
                      frame 4 {
                        w440 = 32  # Hi
                        w441 = 25  # Lo
                        # "Cell 5"
                      }
                    }
                    n195 = global read "Global ER2007.vi" "A/D Pages"() -> (w418:i32[])
                    n196 = global read "Global ER2007.vi" "A/D Volts"() -> (w415:dbl[])
                    n197 = To Single Precision Float(number=w415) -> (single precision float=w404:sgl[])
                    n198 = Index Array(array=w418, index=w417) -> (element=w408:i32)
                    n199 = Index Array(array=w403, index=w408) -> (element=w410:T6)
                    n200 = Index Array(array=w404, index #1=w406, index #2=w405) -> (element #1=w414:sgl, element #2=w413:sgl)
                    n201 = Unbundle By Name(w410) -> ("ChlZero"=w416:sgl[])
                    n202 = Replace Array Subset(array=w416, new element #1=w414, index #1=w412, new element #2=w413, index #2=w411) -> (w409:sgl[])
                    n203 = Bundle By Name(cluster=w410, "ChlZero"=w409) -> (w407:T6)
                    n204 = Replace Array Subset(array=w403, new element=w407, index=w408) -> (w402:T5)
                  }
                }
              }
              frame #2 {
                # "If \"Continue\", updates cal data file and cluster"
                n205 = case shown="True" w446 {
                  tunnel: w445 -> [_ w447]
                  frame False {
                    # "No update"
                  }
                  frame True {
                    # "User wants to update"
                    n206 = global read "Global ER2007.vi" "CalPath"() -> (w448:path)
                    n207 = call "Write Calibration File.vi"("CalDataIn"=w447, "CalFilepath"=w448) -> ()  [unwired: 6 in]
                    n208 = global write "Global ER2007.vi" "CalData"(w447) -> ()
                  }
                }
              }
              frame #3 {
                # "If \"Continue\", small delay to give global CalData\ntime to refresh"
                n209 = case shown="True" w449 {
                  frame False {
                  }
                  frame True {
                    n210 = Wait (ms)(milliseconds to wait=u32 300) -> ()  [unwired: 1 out]
                  }
                }
              }
              frame #4 {
                # "If \"Continue\", previoius small delay before\ntriggering NewCals"
                n211 = case shown="True" w451 {
                  frame False {
                  }
                  frame True {
                    n212 = global write "Global ER2007.vi" "NewCals"(TRUE ("NewCals")) -> ()
                  }
                }
              }
            }
          }
          event "Cancel": Value Change {
            # "Cancel"
            n213 = event-data() -> ("NewVal"=w460:bool)  [unwired: 1 in]
          }
          event "Exit": Value Change {
            # "Exit"
            n214 = event-data() -> ()  [unwired: 1 in, 1 out]
            n215 = case shown="False" w465 {
              tunnel: [w469 TRUE ("T button?")] -> w464
              frame False {
                n216 = property on="Start" class="Bool"() -> ("Strings [4]"=w473:string[])  [unwired: 2 in, 2 out]
                n217 = Index Array(array=w473) -> (element=w472:string)  [unwired: 1 in]
                n218 = Equal?(x=w472, y="Start Test") -> (x = y?=w470:bool)
                n219 = case shown="True" w470 {
                  tunnel: [TRUE ("T button?") w480] -> w469
                  frame False {
                  }
                  frame True {
                    # "New test - see if file exists"
                    n220 = local read "File"() -> (w479:path)
                    n221 = Strip Path(path=w479) -> (stripped path=w478:path, name=w477:string)
                    n222 = call "File Open Logic.vi"("PathIn"=w478, "Filename"=w477, "Auto Append"=TRUE) -> ("AppndOut"=w475:bool)  [unwired: 11 in, 5 out]
                    n223 = case shown="True" w475 {
                      tunnel: [TRUE ("T button?") w482] -> w480
                      frame False {
                        # "File not exist"
                      }
                      frame True {
                        # "File exists"
                        n224 = Two Button Dialog(message="File exists - Continue will append data to existing file", 2:"Continue" ("T button name (\"OK\")")) -> (T button?=w482:bool)  [unwired: 1 in]
                      }
                    }
                  }
                }
              }
              frame True {
              }
            }
            n225 = And(x=w463, y=w464) -> (x .and. y?=→"NewData":bool)
          }
        }
      }
    }
    frame #2 {
      # "Saves, cleanup and shutdown"
      n226 = stacked-sequence {
        tunnel: w495 -> [_ _ _ w615 _ w626]
        tunnel: w494 -> [w500 w587 w612 _ _ _]
        tunnel: w493 -> [w499 _ _ _ _ _]
        tunnel: w492 -> [w498 _ _ _ _ _]
        tunnel: w491 -> [_ _ _ w617 _ _]
        tunnel: w490 -> [_ _ _ w616 _ _]
        tunnel: w489 -> [w497 _ _ _ _ _]
        tunnel: w488 -> [w496 _ _ _ _ _]
        tunnel: w487 -> [_ w586 _ _ _ _]
        tunnel: w486 -> [_ w585 _ _ _ _]
        frame #0 {
          # "Save 1 - updates TestInfo"
          n227 = case shown="True" w500 {
            tunnel: w499 -> [_ w537]
            tunnel: w498 -> [_ w506]
            tunnel: w497 -> [_ w519]
            tunnel: w496 -> [_ w509]
            frame False {
              # "Don't save"
              n228 = global write "Global ER2007.vi" "SUP Cleared"(FALSE ("SUP Cleared")) -> ()
            }
            frame True {
              # "Save"
              # "New"
              # "Prev"
              n229 = local read "Electrode Spacing"() -> (w523:dbl)
              n230 = local read "Acquisition Period"() -> (w525:dbl)
              n231 = Unbundle By Name(w519) -> ("Cell Status"=w534:enum16{"Inactive", "Setup", "Active", "Done"}, "DAQ Period"=w514:u32, "DAQ Units"=w515:u16)
              n232 = Get Date/Time In Seconds() -> (seconds since 1Jan1904=w533:timestamp)
              n233 = To Double Precision Float(number=w533) -> (double precision float=w532:dbl)
              n234 = Unbundle By Name(w519) -> ("Next Time"=w518:dbl)
              n235 = case shown="0, Default" "DAQ Units" {
                tunnel: [w573 w577] -> w512
                tunnel: w525 -> [w575 w579]
                tunnel: [w574 w578] -> w530
                frame 0, Default {
                  # "Mins"
                  n236 = Multiply(x=w575, y=60.0) -> (x*y=w573:dbl)
                  n237 = To Unsigned Long Integer(number=w575) -> (unsigned 32bit integer=w574:u32)
                }
                frame 1 {
                  # "Hrs"
                  n238 = Multiply(x=w579, y=3600.0) -> (x*y=w577:dbl)
                  n239 = To Unsigned Long Integer(number=w579) -> (unsigned 32bit integer=w578:u32)
                }
              }
              n240 = case shown="\"Inactive\", Default" w534 {
                selector: w534 -> [_ w582 w583 _]
                tunnel: [enum16{"Inactive", "Setup", "Active", "Done"}."Setup" ("Cell Status") w582 w583 enum16{"Inactive", "Setup", "Active", "Done"}."Inactive" ("Cell Status")] -> w541
                frame "Inactive", Default {
                }
                frame "Setup" {
                }
                frame "Active" {
                }
                frame "Done" {
                }
              }
              n241 = case shown="0, Default" w515 {
                tunnel: [w550 w554] -> w511
                tunnel: w514 -> [w552 w556]
                tunnel: [w551 w555] -> _
                frame 0, Default {
                  # "Mins"
                  n242 = Multiply(x=w552, y=60.0) -> (x*y=w550:dbl)
                  n243 = To Unsigned Long Integer(number=w552) -> (unsigned 32bit integer=w551:u32)
                }
                frame 1 {
                  # "Hrs"
                  n244 = Multiply(x=w556, y=3600.0) -> (x*y=w554:dbl)
                  n245 = To Unsigned Long Integer(number=w556) -> (unsigned 32bit integer=w555:u32)
                }
              }
              n246 = Not Equal?(x=w511, y=w512) -> (x != y?=w513:bool)
              n247 = case shown="\"Active\"" w534 {
                tunnel: w532 -> [w558 w560 w562 w572]
                tunnel: w518 -> [_ _ w566 _]
                tunnel: w511 -> [_ w559 w564 _]
                tunnel: [w558 w561 w565 w572] -> w517
                tunnel: w512 -> [_ _ w563 _]
                tunnel: w513 -> [_ _ w567 _]
                frame "Inactive", Default {
                }
                frame "Setup" {
                  n248 = Add(x=w559, y=w560) -> (x+y=w561:dbl)
                }
                frame "Active" {
                  n249 = case shown="True" w567 {
                    tunnel: w566 -> [w568 _]
                    tunnel: [w568 w571] -> w565
                    tunnel: w564 -> [_ _]
                    tunnel: w563 -> [_ _]
                    tunnel: w562 -> [_ w570]
                    frame False {
                    }
                    frame True {
                      # "Interval chgd"
                      n250 = Add(x=10.0, y=w570) -> (x+y=w571:dbl)
                    }
                  }
                }
                frame "Done" {
                }
              }
              n251 = local read "Frequency (Hz)"() -> (w524:dbl)
              n252 = local read "Sample ID"() -> (w528:string)
              n253 = local read "Length"() -> (w521:dbl)
              n254 = local read "Fluid Pair"() -> (w526:string)
              n255 = global read "Global ER2007.vi" "Test Info"() -> (w508:T2)
              n256 = local read "Project"() -> (w529:string)
              n257 = global read "Global ER2007.vi" "DefExcAmplt"() -> (w507:dbl)
              n258 = local read "Rock Type"() -> (w527:string)
              n259 = local read "Diameter"() -> (w522:dbl)
              n260 = local read "File"() -> (w520:path)
              n261 = case shown="\"Lo Range\"" "PoreXdcr" {
                tunnel: [enum16{"<none>", "Lo Range", "Hi Range"}."Lo Range" ("Last Pore Xdcr") enum16{"<none>", "Lo Range", "Hi Range"}."Hi Range" ("Last Pore Xdcr")] -> w505
                frame "Lo Range" {
                }
                frame "Hi Range", Default {
                }
              }
              n262 = Unbundle By Name(w508) -> ("Cell Data"=w510:T3)
              n263 = case shown="0, Default" "4P/2P" {
                tunnel: [FALSE TRUE] -> w502
                frame 0, Default {
                }
                frame 1 {
                }
              }
              n264 = Bundle By Name(cluster=w519, "Cell ID"=w506, "Cell Status"=w541, "Project"=w529, "Sample #"=w528, "Rock Type"=w527, "Fluid Pair"=w526, "Rw"="Rw", "Rw Temp"="Rw_Temp", "Length"=w521, "Diameter"=w522, "Porosity"="Porosity", "Permeability"="Permeability", "ElectSpace"=w523, "Frequency"=w524, "Amplitude"=w507, "DAQ Period"=w530, "DAQ Units"="DAQ Units", "Datafile"=w520, "Next Time"=w517, "Last Pore Xdcr"=w505, "4P"=w502) -> (w538:T4)
              n265 = Replace Array Subset(array=w510, new element=w538, index=w537) -> (w536:T3)
              n266 = case shown="True" w509 {
                tunnel: w536 -> [_ w549]
                tunnel: w506 -> [_ w548]
                tunnel: w508 -> [_ w547]
                frame False {
                }
                frame True {
                  n267 = Bundle By Name(cluster=w547, "CurCell"=w548, "Cell Data"=w549) -> (w546:T2)
                  n268 = global write "Global ER2007.vi" "Test Info"(w546) -> ()
                }
              }
              n269 = global write "Global ER2007.vi" "SupStatusCell"(w506) -> ()
            }
          }
        }
        frame #1 {
          # "Save 2 - updates NoGalil global and defaults file"
          n270 = case shown="True" w587 {
            tunnel: w586 -> [_ w590]
            tunnel: w585 -> [_ w588]
            frame False {
              # "Don't save"
            }
            frame True {
              # "Save"
              n271 = Not Equal?(x=w590, y=w588) -> (x != y?=w589:bool)
              n272 = case shown="True" w589 {
                tunnel: w588 -> [_ w595]
                frame False {
                }
                frame True {
                  # "Reads the Defaults file and updates it with\nthe new \"No Galil\" global"
                  n273 = global read "Global ER2007.vi" "Defaults Filename"() -> (w611:string)
                  n274 = global write "Global ER2007.vi" "No Galil"(w595) -> ()
                  n275 = call "Read Defaults File.vi"("Filename"=w611) -> ("DirPath3"=w608:path, "DirPath2"=w609:path, "DirPath1"=w610:path, "DirPath4"=w607:path, "DirPath5"=w606:path, "String1"=w605:string, "String2"=w604:string, "String3"=w603:string, "String4"=w602:string, "MiscPath1"=w599:path, "String5"=w601:string, "BooleanArray"=w598:bool[], "IntegerArray1"=w594:i32[], "IntegerArray2"=w593:i32[], "RealArray1"=w592:dbl[], "RealArray2"=w591:dbl[], "StringArray"=w600:string[])  [unwired: 10 out]
                  n276 = Replace Array Subset(array=w598, new element=w595, index=10) -> (w597:bool[])
                  n277 = call "Write Defaults File.vi"("DirPath3"=w608, "DirPath2"=w609, "DirPath1"=w610, "DefaultFilename"=w611, "DirPath4"=w607, "DirPath5"=w606, "String1"=w605, "String2"=w604, "String3"=w603, "String4"=w602, "MiscPath1"=w599, "String5"=w601, "BooleanArray"=w597, "IntegerArray1"=w594, "IntegerArray2"=w593, "RealArray1"=w592, "RealArray2"=w591, "StringArray"=w600) -> ()  [unwired: 10 in]
                }
              }
            }
          }
        }
        frame #2 {
          # "Save 3 - sets global Setup flags"
          n278 = case shown="True" w612 {
            frame False {
              # "Don't save"
            }
            frame True {
              w613 = TRUE ("New Setup")
              # "Save"
              n279 = global write "Global ER2007.vi" "New Sup Status"(w613) -> ()
              n280 = global write "Global ER2007.vi" "New Setup"(w613) -> ()
            }
          }
        }
        frame #3 {
          w614 = u8 0 ("Disabled")
          # "Clears visable properties; opens front panel of calling vi before returning"
          n281 = case shown="True" w615 {
            tunnel: w616 -> [_ w618]
            tunnel: w617 -> [_ w619]
            frame False {
            }
            frame True {
              # "Opens and returns to Test Panel"
              n282 = property class="VI"(reference=w618, error in=w619, "Front Panel Window:Open"=TRUE) -> (reference out=w622:refnum<vi>, error out=w621:errorcluster)
              n283 = Close Reference(reference=w622, error in (no error)=w621) -> (error out=w620:errorcluster)
              n284 = call <vilib>:"Simple Error Handler.vi"("error in (no error)"=w620) -> ()  [unwired: 4 in, 5 out]
            }
          }
          n285 = property on="Project" class="Str"("Disabled"=w614) -> ()  [unwired: 2 in, 2 out]
          n286 = property on="Length" class="DigNum (strict)"("Disabled"=w614) -> ()  [unwired: 2 in, 2 out]
          n287 = property on="Start" class="Bool"("Disabled"=w614) -> ()  [unwired: 2 in, 2 out]
          n288 = property on="Diameter" class="DigNum (strict)"("Disabled"=w614) -> ()  [unwired: 2 in, 2 out]
          n289 = property on="Sample ID" class="Str"("Disabled"=w614) -> ()  [unwired: 2 in, 2 out]
          n290 = property on="Stop" class="Bool"("Disabled"=w614) -> ()  [unwired: 2 in, 2 out]
          n291 = property on="Porosity" class="DigNum (strict)"("Disabled"=w614) -> ()  [unwired: 2 in, 2 out]
          n292 = property on="Clear" class="Bool"("Disabled"=w614) -> ()  [unwired: 2 in, 2 out]
          n293 = property on="Rock Type" class="Str"("Disabled"=w614) -> ()  [unwired: 2 in, 2 out]
          n294 = property on="Permeability" class="DigNum (strict)"("Disabled"=w614) -> ()  [unwired: 2 in, 2 out]
          n295 = property on="Exit" class="Bool"("Disabled"=w614) -> ()  [unwired: 2 in, 2 out]
          n296 = property on="Fluid Pair" class="Str"("Disabled"=w614) -> ()  [unwired: 2 in, 2 out]
          n297 = property on="Electrode Spacing" class="DigNum (strict)"("Disabled"=w614) -> ()  [unwired: 2 in, 2 out]
          n298 = property on="ZeroPore" class="Bool"("Disabled"=w614) -> ()  [unwired: 2 in, 2 out]
          n299 = property on="Rw" class="DigNum (strict)"("Disabled"=w614) -> ()  [unwired: 2 in, 2 out]
          n300 = property on="Rw_Temp" class="DigNum (strict)"("Disabled"=w614) -> ()  [unwired: 2 in, 2 out]
          n301 = property on="Volume Measurement" class="Ring (strict)"("Disabled"=w614) -> ()  [unwired: 2 in, 2 out]
          n302 = property on="File" class="Path"("Disabled"=w614) -> ()  [unwired: 2 in, 2 out]
          n303 = property on="Frequency (Hz)" class="DigNum (strict)"("Disabled"=w614) -> ()  [unwired: 2 in, 2 out]
        }
        frame #4 {
          n304 = Wait (ms)(milliseconds to wait=u32 500) -> ()  [unwired: 1 out]
        }
        frame #5 {
          # "All done - close this panel"
          n305 = case shown="True" w626 {
            frame False {
            }
            frame True {
              # "Close this panel's front panel"
              n306 = Current VI's Path() -> (path=w633:path)
              n307 = Open VI Reference(vi path=w633) -> (vi reference=w632:refnum<vi>, error out=w631:errorcluster)  [unwired: 5 in]
              n308 = property class="VI"(reference=w632, error in=w631, "Front Panel Window:Open"=FALSE) -> (reference out=w629:refnum<vi>, error out=w628:errorcluster)
              n309 = Close Reference(reference=w629, error in (no error)=w628) -> (error out=w627:errorcluster)
              n310 = call <vilib>:"Simple Error Handler.vi"("error in (no error)"=w627) -> ()  [unwired: 4 in, 5 out]
            }
          }
          n311 = global write "Global ER2007.vi" "SUP Done"(TRUE ("SUP Done")) -> ()
        }
      }
    }
  }
